vi "AddHelper.vi"(8 "error in (no error)":errorcluster, 9 "Helper Name":string, 10 "Module Name":string, 11 "Module Ref":refnum<vi>) -> (0 "error out":errorcluster)   [LabVIEW 2024, in "AddHelper.lvlib"]
uses:
  AddHelper.lvlib
  <vilib>/Utility/traverseref.llb/TRef TravTarget.ctl
  <vilib>/Utility/traverseref.llb/VI Scripting - Traverse.lvlib
  <vilib>/Utility/miscctls.llb/LVPointTypeDef.ctl
  templates/HelperTemplate.vi
  <vilib>/Utility/Data Type/NI_Data Type.lvlib
  <vilib>/event_ctls.llb/lveventtype.ctl
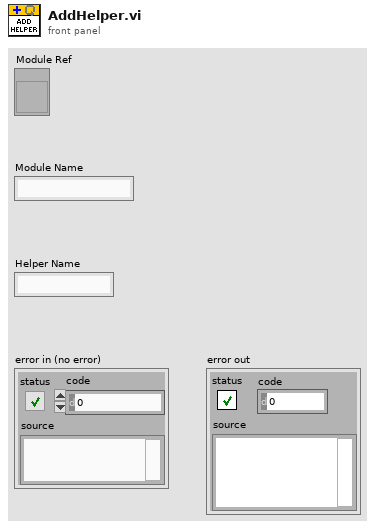
[diagram p1: front panel]
types:
  T1 = typedef "lveventtype.ctl" = enum32{"Null", "Timeout", "Annotation Menu Selection", "Annotation Menu Selection?", "App Instance Close", "App Instance Close?", "Autoscale Range Change", "Bookmark Info Change", "Cell Edit", "Cell Edit?", "Cursor Grab", "Cursor Grab?", "Cursor Menu Selection", "Cursor Menu Selection?", "Cursor Move", "Cursor Release", "Data Change", "Direction Change", "Display State Change", "Drag Ended", "Drag Enter", "Drag Leave", "Drag Over", "Drag Source Update", "Drag Starting", "Drag Starting?", "Drop", "Exec State Change", "Key Down", "Key Down?", "Key Repeat", "Key Repeat?", "Key Up", "Listbox Double Click", "Menu Activation?", "Menu Selection (App)", "Menu Selection? (App)", "Menu Selection (User)", "Mouse Down", "Mouse Down?", "Mouse Enter", "Mouse Leave", "Mouse Move", "Mouse Up", "Mouse Wheel", "NI Security User Change (App)", "Pane Size", "Panel Close", "Panel Close?", "Panel Resize", "Plot Attribute Change", "Scale Range Change", "Shortcut Menu Activation?", "Shortcut Menu Selection (App)", "Shortcut Menu Selection? (App)", "Shortcut Menu Selection (User)", "Tree Double Click", "Tree Drag", "Tree Drag?", "Tree Drop", "Tree Drop?", "Tree Item Close", "Tree Item Close?", "Tree Item Open", "Tree Item Open?", "User Event", "Value Change"}
  T2 = cluster{"Event Type":T1, "Event Registration Index":i32}[]
  T3 = typedef "TRef TravTarget.ctl" = enum16{"FP", "BD", "Other"}
  T4 = typedef "LVPointTypeDef.ctl" = cluster{"Horizontal":i16, "Vertical":i16}
  T5 = typedef "LVPositionTypeDef.ctl" = cluster{"Left":i32, "Top":i32}
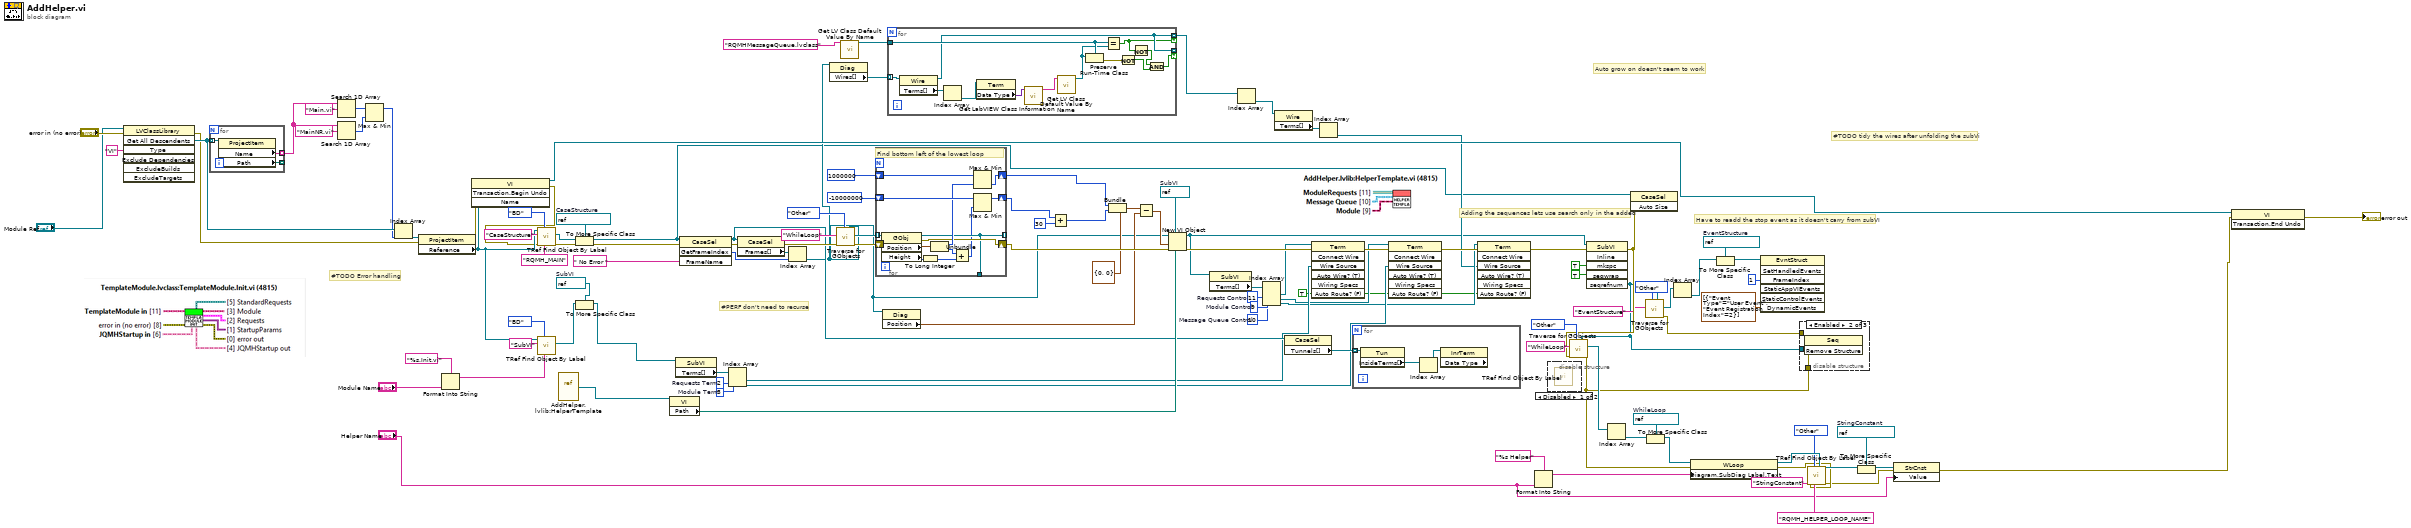
[diagram p0: block diagram]
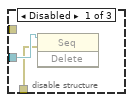
[diagram p2: hidden frame]
diagram:
  w6 = refnum<vi> refnum  # EventStructure
  w18 = refnum<vi> refnum  # StringConstant
  w29 = refnum<vi> refnum  # WhileLoop
  w54 = 10  # Message Queue Control
  w38 = TRUE ("Auto Route? (F)")
  w57 = 9  # Module Control
  w61 = 11  # Requests Control
  w63 = 3  # Module Term
  w64 = 2  # Requests Term
  w66 = refnum<vi> refnum  # SubVI
  w87 = refnum<vi> refnum  # SubVI
  w100 = refnum<vi> refnum  # CaseStructure
  # "Have to readd the stop event as it doesn't carry from subVI"
  # "#TODO tidy the wires after unfolding the subVi"
  # "Adding the sequences lets use search only in the added"
  # "Auto grow on doesn't seem to work"
  # "#PERF don't need to recurse"
  # "#TODO Error handling"
  n1 = invoke class="LVClassLibrary" method="Get All Descendents"(reference="Module Ref", error in="error in (no error)", "Type"="VI") -> (error out=w108:errorcluster, "All Descendents"=w111:refnum<vi>[])  [unwired: 4 in, 5 out]
  n2 = for {
    tunnel: w111 -> [w120] mode=indexing
    tunnel: [w119] -> w112 mode=indexing
    tunnel: [w118] -> _ mode=indexing
    n3 = property class="ProjectItem"(reference=w120) -> ("Name"=w119:string, "Path"=w118:path)  [unwired: 1 in, 2 out]
  }
  n4 = Search 1D Array(1D array=w112, element="Main.vi") -> (index of element=w114:i32)  [unwired: 1 in]
  n5 = Search 1D Array(1D array=w112, element="MainNR.vi") -> (index of element=w113:i32)  [unwired: 1 in]
  n6 = Max & Min(x=w114, y=w113) -> (max(x,y)=w109:i32)  [unwired: 1 out]
  n7 = Index Array(array=w111, index=w109) -> (element=w110:refnum<vi>)
  n8 = property class="ProjectItem"(reference=w110, error in=w108) -> (error out=w47:errorcluster, "Reference"=w48:refnum<vi>)  [unwired: 1 out]
  n9 = Format Into String(format string="%s.Init.vi", "Module Name") -> (resulting string=w71:string)  [unwired: 2 in, 1 out]
  n10 = invoke class="VI" method="Transaction.Begin Undo"(reference=w48, error in=w47) -> (reference out=w45:refnum<vi>, error out=w46:errorcluster)  [unwired: 2 in, 2 out]
  n11 = call <vilib>:"TRef Find Object By Label.vi"("Label"="RQMH_MAIN", "Traverse Target"=TRef_TravTarget."BD", "error in (no error)"=w46, "Class Name"="CaseStructure", "VI Ref"=w48) -> ("error out"=w102:errorcluster, "Found Obj Ref"=w101:refnum<vi>)  [unwired: 3 in, 2 out]
  n12 = call <vilib>:"TRef Find Object By Label.vi"("Label"=w71, "Traverse Target"=TRef_TravTarget."BD", "Class Name"="SubVI", "VI Ref"=w48) -> ("Found Obj Ref"=w68:refnum<vi>)  [unwired: 4 in, 3 out]
  n13 = vi-ref "AddHelper.lvlib:HelperTemplate.vi"() -> (w78:refnum<vi>)
  n14 = To More Specific Class(target class=w100, reference=w101, error in=w102) -> (specific class reference=w34:refnum<vi>, error out=w33:errorcluster)
  n15 = To More Specific Class(target class=w66, reference=w68) -> (specific class reference=w67:refnum<vi>)  [unwired: 1 in, 1 out]
  n16 = property class="VI"(reference=w78) -> ("Path"=w77:path)  [unwired: 1 in, 2 out]
  n17 = property class="SubVI"(reference=w67) -> ("Terms[]"=w65:refnum<vi>[])  [unwired: 1 in, 2 out]
  n18 = invoke class="CaseSel" method="GetFrameIndex"(reference=w34, error in=w33, "FrameName"=" No Error " ("Frame Name")) -> (reference out=w75:refnum<vi>, error out=w98:errorcluster, "GetFrameIndex"=w96:i32)  [unwired: 1 in, 1 out]
  n19 = Index Array(array=w65, index #1=w64, index #2=w63) -> (element #1=w59:refnum<vi>, element #2=w55:refnum<vi>)
  n20 = property class="CaseSel"(reference=w75, error in=w98) -> (error out=w95:errorcluster, "Frames[]"=w97:refnum<vi>[])  [unwired: 1 out]
  n21 = Index Array(array=w97, index=w96) -> (element=w43:refnum<vi>)
  n22 = property class="Diag"(reference=w43) -> ("Wires[]"=w42:refnum<vi>[])  [unwired: 1 in, 2 out]
  n23 = call <vilib>:"Traverse for GObjects.vi"("Other Refnum"=w43, "Traverse Target"=TRef_TravTarget."Other", "error in (no error)"=w95, "Class Name"="WhileLoop") -> ("error out"=w89:errorcluster, "References"=w92:refnum<vi>[])  [unwired: 4 in, 2 out]
  n24 = call <vilib>:"Get LV Class Default Value By Name.vi"("class name"="RQMHMessageQueue.lvclass") -> ("object"=w40:refnum<class>)  [unwired: 9 in, 1 out]
  n25 = for {
    tunnel: w92 -> [w134] mode=indexing
    tunnel: [w126] -> _ mode=indexing
    shift-right: [w130] -> w82
    shift-left: 1000000 ("Left") -> [w132]
    shift-right: [w125] -> w81
    shift-left: -10000000 ("Left") -> [w131]
    shift-right: [w127] -> w88
    shift-left: w89 -> [w128]
    tunnel: [w126] -> _
    # "Find bottom left of the lowest loop"
    n26 = property class="GObj"(reference=w134, error in=w128) -> (reference out=w126:refnum<vi>, error out=w127:errorcluster, "Position"=w133:T5, "Height"=w123:u32)
    n27 = To Long Integer(number=w123) -> (32bit integer=w121:i32)
    n28 = Unbundle(w133) -> ("Left"=w129:i32, "Top"=w124:i32)
    n29 = Add(x=w124, y=w121) -> (x+y=w122:i32)
    n30 = Max & Min(x=w132, y=w129) -> (min(x,y)=w130:i32)  [unwired: 1 out]
    n31 = Max & Min(x=w131, y=w122) -> (max(x,y)=w125:i32)  [unwired: 1 out]
  }
  n32 = property class="Diag"(reference=w43) -> ("Position"=w84:T5)  [unwired: 1 in, 2 out]
  n33 = for {
    tunnel: w42 -> [w147] mode=indexing
    tunnel: w40 -> [w141]
    tunnel: [w139] -> w39 mode=indexing if=w138
    tunnel: [w139] -> _ mode=indexing if=w135
    n34 = property class="Wire"(reference=w147) -> (reference out=w139:refnum<vi>, "Terms[]"=w146:refnum<vi>[])  [unwired: 1 in, 1 out]
    n35 = Index Array(array=w146) -> (element=w145:refnum<vi>)  [unwired: 1 in]
    n36 = property class="Term"(reference=w145) -> ("Data Type"=w144:variant)  [unwired: 1 in, 2 out]
    n37 = call <vilib>:"Get LabVIEW Class Information.vi"("variant"=w144) -> ("LabVIEW class file name"=w143:string)  [unwired: 8 in, 2 out]
    n38 = call <vilib>:"Get LV Class Default Value By Name.vi"("class name"=w143) -> ("object"=w140:refnum<class>)  [unwired: 9 in, 1 out]
    n39 = Preserve Run-Time Class(object in=w140, 2:w141) -> (error out=w142:errorcluster)  [unwired: 1 in, 1 out]
    n40 = Equal?(x=w141, y=w140) -> (x = y?=w138:bool)
    n41 = Not(x=w142) -> (.not. x?=w137:bool)
    n42 = Not(x=w138) -> (.not. x?=w136:bool)
    n43 = And(x=w136, y=w137) -> (x .and. y?=w135:bool)
  }
  n44 = Add(x=w81, y=30) -> (x+y=w79:i32)
  n45 = Bundle(cluster=T4 {"Horizontal"=0, "Vertical"=0} ("location"), "Horizontal"=w82, "Vertical"=w79) -> (w85:T4)
  n46 = Subtract(x=w85, y=w84) -> (x-y=w83:T5)
  n47 = New VI Object(vi object class=w87, owner refnum=w43, position/next to=w83, 6:w77, 8:w88) -> (object refnum=w32:refnum<vi>, 0:w76:errorcluster)  [unwired: 3 in]
  n48 = property class="SubVI"(reference=w32) -> ("Terms[]"=w62:refnum<vi>[])  [unwired: 1 in, 2 out]
  n49 = Index Array(array=w39) -> (element=w36:refnum<vi>)  [unwired: 1 in]
  n50 = Index Array(array=w62, index #1=w61, index #2=w57, index #3=w54) -> (element #1=w60:refnum<vi>, element #2=w56:refnum<vi>, element #3=w50:refnum<vi>)
  n51 = property class="Wire"(reference=w36) -> ("Terms[]"=w37:refnum<vi>[])  [unwired: 1 in, 2 out]
  n52 = property class="CaseSel"(reference=w75) -> ("Tunnels[]"=w74:refnum<vi>[])  [unwired: 1 in, 2 out]
  n53 = invoke class="Term" method="Connect Wire"(reference=w60, error in=w76, "Wire Source"=w59, "Auto Route? (F)"=w38) -> (error out=w58:errorcluster)  [unwired: 3 in, 6 out]
  n54 = Index Array(array=w37) -> (element=w35:refnum<vi>)  [unwired: 1 in]
  n55 = for {
    tunnel: w74 -> [w150] mode=indexing
    n56 = property class="Tun"(reference=w150) -> ("InsideTerms[]"=w149:refnum<vi>[])  [unwired: 1 in, 2 out]
    n57 = Index Array(array=w149) -> (element=w148:refnum<vi>)  [unwired: 1 in]
    n58 = property class="InrTerm" props=["Data Type"](reference=w148) -> ()  [unwired: 1 in, 3 out]
  }
  n59 = invoke class="Term" method="Connect Wire"(reference=w56, error in=w58, "Wire Source"=w55, "Auto Route? (F)"=w38) -> (error out=w51:errorcluster)  [unwired: 3 in, 6 out]
  n60 = invoke class="Term" method="Connect Wire"(reference=w50, error in=w51, "Wire Source"=w35, "Auto Route? (F)"=w38) -> (error out=w49:errorcluster)  [unwired: 3 in, 6 out]
  n61 = Format Into String(format string="%s Helper", "Helper Name") -> (resulting string=w24:string)  [unwired: 2 in, 1 out]
  n62 = disable-structure shown="Disabled" {
    frame Disabled {
      n63 = call <vilib>:"TRef Find Object By Label.vi"() -> ()  [unwired: 8 in, 4 out]
    }
    frame Enabled {
    }
  }
  n64 = invoke class="SubVI" method="Inline"(reference=w32, error in=w49, "mkspc"=TRUE ("Make Space in Block Diagram"), "seqwrap"=TRUE ("Wrap in Sequence")) -> (error out=w11:errorcluster, "seqrefnum"=w9:refnum<vi>)  [unwired: 2 in, 4 out]
  n65 = call <vilib>:"Traverse for GObjects.vi"("Other Refnum"=w9, "Traverse Target"=TRef_TravTarget."Other", "error in (no error)"=w11, "Class Name"="WhileLoop") -> ("error out"=w12:errorcluster, "References"=w28:refnum<vi>[])  [unwired: 4 in, 2 out]
  n66 = Index Array(array=w28) -> (element=w27:refnum<vi>)  [unwired: 1 in]
  n67 = invoke class="CaseSel" method="Auto Size"(reference=w34, error in=w11) -> ()  [unwired: 1 in, 3 out]
  n68 = call <vilib>:"Traverse for GObjects.vi"("Other Refnum"=w9, "Traverse Target"=TRef_TravTarget."Other", "Class Name"="EventStructure") -> ("error out"=w7:errorcluster, "References"=w2:refnum<vi>[])  [unwired: 5 in, 2 out]
  n69 = To More Specific Class(target class=w29, reference=w27) -> (specific class reference=w26:refnum<vi>)  [unwired: 1 in, 1 out]
  n70 = Index Array(array=w2) -> (element=w1:refnum<vi>)  [unwired: 1 in]
  n71 = property class="WLoop"(reference=w26, error in=w12, "Diagram.SubDiag Label.Text"=w24) -> (reference out=w22:refnum<vi>, error out=w15:errorcluster)
  n72 = To More Specific Class(target class=w6, reference=w1) -> (specific class reference=w5:refnum<vi>)  [unwired: 1 in, 1 out]
  n73 = invoke class="EvntStruct" method="SetHandledEvents"(reference=w5, "FrameIndex"=1 ("Frame Index"), "DynamicEvents"=T2 [{"Event Type"=enum."User Event", "Event Registration Index"=2}] ("Dynamic Events")) -> ()  [unwired: 4 in, 7 out]
  n74 = disable-structure shown="Enabled" {
    disable-tunnel: w9 -> [w152 w154 _]
    disable-tunnel: w12 -> [w151 w153 _]
    disable-tunnel: w7 -> [_ _ _]
    frame Disabled {
      n75 = invoke class="Seq" method="Delete"(reference=w152, error in=w151) -> ()  [unwired: 1 in, 3 out]
    }
    frame Enabled {
      n76 = invoke class="Seq" method="Remove Structure"(reference=w154, error in=w153) -> ()  [unwired: 1 in, 3 out]
    }
    frame Disabled {
    }
  }
  n77 = call <vilib>:"TRef Find Object By Label.vi"("Other Refnum"=w22, "Label"="RQMH_HELPER_LOOP_NAME", "Traverse Target"=TRef_TravTarget."Other", "error in (no error)"=w15, "Class Name"="StringConstant") -> ("error out"=w14:errorcluster, "dup VI Ref"=w19:refnum<vi>)  [unwired: 3 in, 2 out]
  n78 = To More Specific Class(target class=w18, reference=w19) -> (specific class reference=w17:refnum<vi>)  [unwired: 1 in, 1 out]
  n79 = property class="StrCnst"(reference=w17, error in=w14, "Value"="Helper Name") -> (error out=w13:errorcluster)  [unwired: 1 out]
  n80 = invoke class="VI" method="Transaction.End Undo"(reference=w45, error in=w13) -> (error out=→"error out":errorcluster)  [unwired: 1 in, 2 out]
